vi "DequeueElement.vi"(9 "Logging Data?":refnum<vi>, 10 "Data Queue":refnum<vi>, 11 "File Connection Refnum":refnum<file>) -> (1 "# elements in queue":i32, 3 "File Connection Out":refnum<file>)   [LabVIEW 2021]
panel:
  in  "File Connection":refnum<vi>
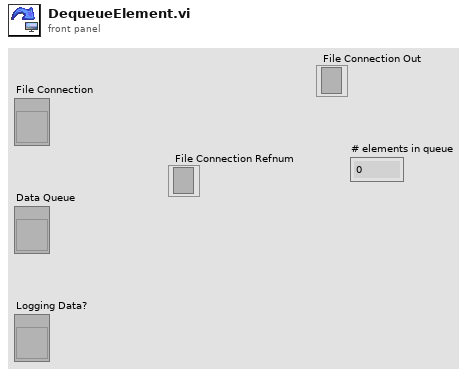
[diagram p1: front panel]
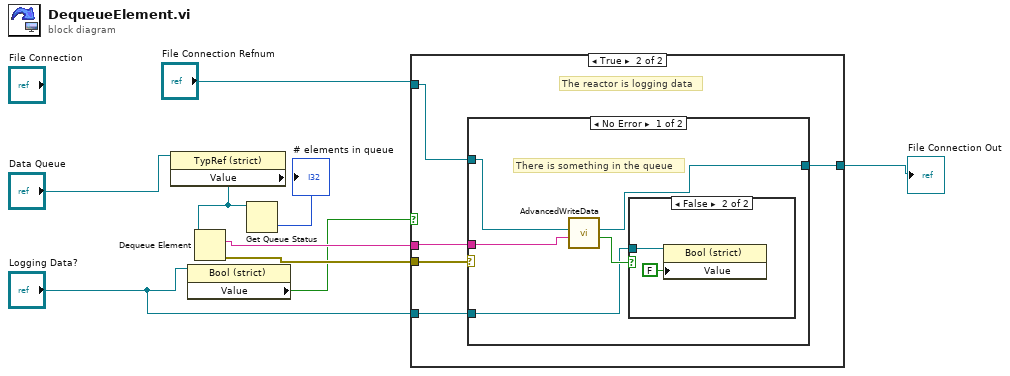
[diagram p0: block diagram]
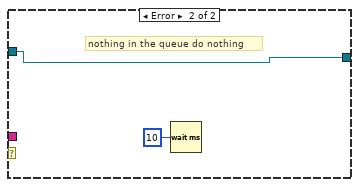
[diagram p4: hidden frame]
diagram:
  n1 = property class="TypRef (strict)"(reference="Data Queue") -> ("Value"=w2:refnum<queue>)  [unwired: 1 in, 2 out]
  n2 = property class="Bool (strict)"(reference="Logging Data?") -> ("Value"=w5:bool)  [unwired: 1 in, 2 out]
  n3 = Dequeue Element(queue=w2) -> (element=w7:string, error out=w6:errorcluster)  [unwired: 2 in, 2 out]
  n4 = Get Queue Status(queue=w2) -> (# elements in queue=→"# elements in queue":i32)  [unwired: 2 in, 7 out]
  n5 = case shown="True" w5 {
    tunnel: w7 -> [_ w15]
    tunnel: "Logging Data?" -> [_ w14]
    tunnel: w6 -> [_ w13]
    tunnel: [w10 w12] -> w4
    tunnel: "File Connection Refnum" -> [w10 w11]
    frame False {
      # "reactor is not logging data do not write the pressure"
    }
    frame True {
      # "The reactor is logging data"
      n6 = case shown="No Error" w13 {
        tunnel: w15 -> [w20 _]
        tunnel: w14 -> [w18 _]
        tunnel: [w17 w24] -> w12
        tunnel: w11 -> [w16 w24]
        frame No Error {
          # "There is something in the queue"
          n7 = call "AdvancedWriteData.vi"("Data String"=w20, "File Connection"=w16) -> ("Sucessful?"=w19:bool, "File Connection Out"=w17:refnum<file>)  [unwired: 8 in]
          n8 = case shown="False" w19 {
            tunnel: w18 -> [_ w22]
            frame True {
            }
            frame False {
              n9 = property class="Bool (strict)"(reference=w22, "Value"=FALSE) -> ()  [unwired: 1 in, 2 out]
            }
          }
        }
        frame Error {
          # "nothing in the queue do nothing"
          n10 = Wait (ms)(milliseconds to wait=u32 10) -> ()  [unwired: 1 out]
        }
      }
    }
  }
  "File Connection Out" <- w4
